vi "GLOBALVision.vi"() -> ()   [LabVIEW 2011]
uses:
  <vilib>/Rock Robotics/WPI/Camera/WPI_CameraImageSize.ctl
  <vilib>/Rock Robotics/WPI/Camera/WPI_CameraWhite Balance Values.ctl
  <vilib>/Rock Robotics/WPI/Camera/WPI_CameraExposure Values.ctl
panel:
  in  "Enable Vision":bool
  in  "Camera Settings":T4={"fps"=15, "compression"=30, "Image Size"=enum."640x480", "Camera Resolultion"=[{640, 480}, {320, 240}, {160, 120}], "White Balance"=enum."Fixed fluorescent 1", "Exposure"=enum."Flicker-free 60 Hz", "Brightness"=30.0, "Enable Color"=FALSE, "Camera Address"="10.0.27.11"}
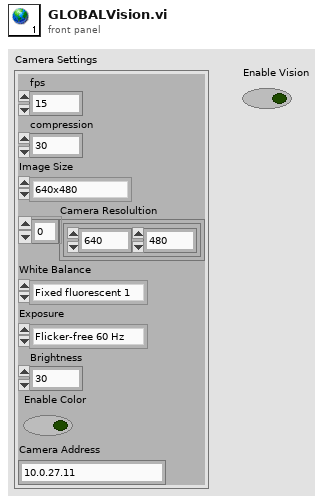
[diagram p1: front panel]
types:
  T1 = typedef "WPI_CameraImageSize.ctl" = enum16{"640x480", "320x240", "160x120"}
  T2 = typedef "WPI_CameraWhite Balance Values.ctl" = enum16{"Auto", "Fixed indoor", "Fixed outdoor 1", "Fixed outdoor 2", "Fixed fluorescent 1", "Fixed fluorescent 2", "Hold current"}
  T3 = typedef "WPI_CameraExposure Values.ctl" = enum16{"Auto", "Flicker-free 50 Hz", "Flicker-free 60 Hz", "Hold current"}
  T4 = cluster{"fps":i32, "compression":i32, "Image Size":T1, "Camera Resolultion":cluster{i32, i32}[], "White Balance":T2, "Exposure":T3, "Brightness":dbl, "Enable Color":bool, "Camera Address":string}
diagram:
